vi "Begin.vi"() -> (0 "error out":errorcluster)   [LabVIEW 2018]
doc: "Called before other user functions, this VI is expected to open initial I/O refnums, load in file data, and do all program initialization. Notice that the <B>error out</B> terminal is simply used for data flow. Wiring it to other structures or subVIs ensures that this VI runs first."
uses:
  <vilib>/Rock Robotics/WPI/DriverStation/WPI_DriverStationRobotMode2.ctl
  <vilib>/Rock Robotics/WPI/Joystick/WPI_JoystickDeviceEnum.ctl
  dsdata.vi
  <vilib>/Rock Robotics/WPI/Utilities/WPI_GetSetVariantRefNum.vi
  refnums.vi
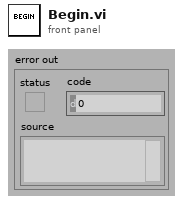
[diagram p1: front panel]
types:
  T1 = typedef "WPI_JoystickDeviceEnum.ctl" = enum16{"USB 0", "USB 1", "USB 2", "USB 3", "USB 4", "USB 5"}
  T2 = typedef "WPI_DriverStationRobotMode2.ctl" = enum16{"Autonomous Disabled", "Autonomous Enabled", "Teleop Disabled", "Teleop Enabled", "Disconnected", "Finish", "Test Disabled", "Test Enabled", "Emergency Stopped"}
  T3 = typedef "WPI_JoystickDevRef.ctl" = cluster{"Device":T1}
  T4 = typedef "WPI_CompressorDevRef.ctl" = cluster{"DevStatus":errorcluster, "Pneumatics Control Module":u8}
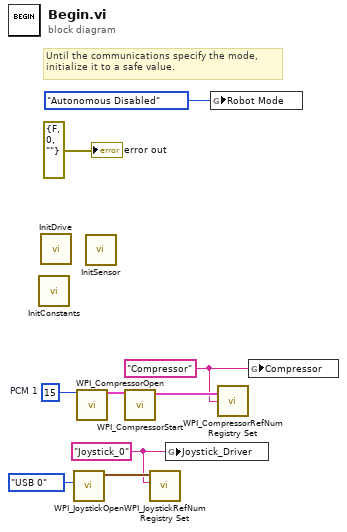
[diagram p0: block diagram]
diagram:
  w1 = "Joystick_0" ("Joystick_0")
  w4 = "Compressor" ("refnum name")
  w6 = u8 15  # PCM 1
  # "Until the communications specify the mode,\ninitialize it to a safe value."
  n1 = call "InitConstants.vi"() -> ()  [unwired: 12 in]
  n2 = call "InitDrive.vi"() -> ()  [unwired: 1 in]
  n3 = call <vilib>:"WPI_JoystickOpen.vi"("JoystickDevice"=WPI_JoystickDeviceEnum."USB 0") -> ("JoystickDevRef"=w2:T3)  [unwired: 10 in]
  n4 = call <vilib>:"WPI_CompressorOpen.vi"("Pneumatics Control Module (0)"=w6) -> ("CompressorDevRef"=w7:T4)  [unwired: 13 in, 1 out]
  n5 = call "InitSensor.vi"() -> ()  [unwired: 1 in]
  n6 = call <vilib>:"WPI_CompressorStart.vi"("CompressorDevRef"=w7) -> ("CompressorDevRef"=w5:T4)  [unwired: 9 in, 1 out]
  n7 = call <vilib>:"WPI_JoystickRefNum Registry Set.vi"("refnum name"=w1, "JoystickDevRef"=w2) -> ()  [unwired: 8 in, 2 out]
  n8 = global write "refnums.vi" "Joystick_Driver"(w1) -> ()
  n9 = global write "dsdata.vi" "Robot Mode"(WPI_DriverStationRobotMode2."Autonomous Disabled" ("Robot Mode")) -> ()
  n10 = call <vilib>:"WPI_CompressorRefNum Registry Set.vi"("refnum name"=w4, "CompressorDevRef"=w5) -> ()  [unwired: 8 in, 2 out]
  n11 = global write "refnums.vi" "Compressor"(w4) -> ()
  "error out" <- errorcluster {"status"=FALSE, "code"=0, "source"=""} ("error in")
